vi "ToggleIndicator.vi"(11 "cClimbWeight":bool) -> (2 "True":bool, 3 "False":bool)   [LabVIEW 2013]
uses:
  ToggleStates.ctl
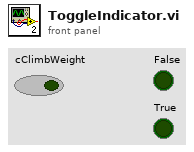
[diagram p1: front panel]
types:
  T1 = typedef "ToggleStates.ctl" = enum16{"Retract2", "Actuate1", "Actuate2", "Retract1"}
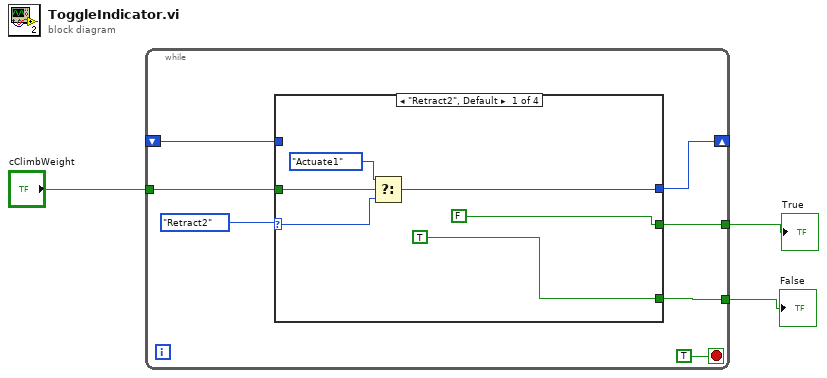
[diagram p0: block diagram]
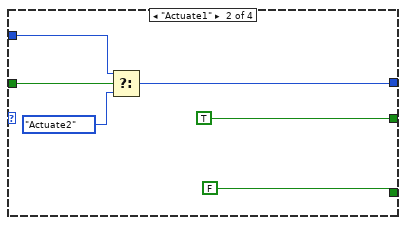
[diagram p2: hidden frame]
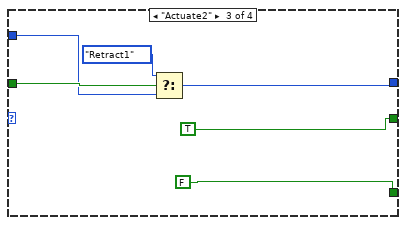
[diagram p3: hidden frame]
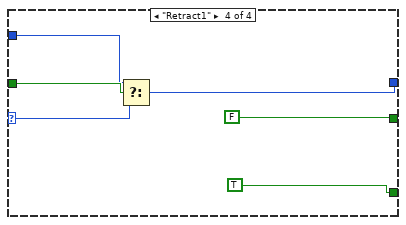
[diagram p4: hidden frame]
diagram:
  n1 = while {
    tunnel: "cClimbWeight" -> [w8]
    shift-right: [w7] -> _
    shift-left: _ -> [w6]
    tunnel: [w5] -> w2
    tunnel: [w4] -> w1
    stop <- TRUE stop-if-true
    n2 = case shown="\"Retract2\", Default" ToggleStates."Retract2" ("Enum") {
      selector: ToggleStates."Retract2" ("Enum") -> [w15 _ _ w29]
      tunnel: w8 -> [w16 w22 w28 w32]
      tunnel: [w13 w20 w23 w30] -> w7
      tunnel: w6 -> [_ w19 w25 w31]
      tunnel: [FALSE TRUE TRUE FALSE] -> w5
      tunnel: [TRUE FALSE FALSE TRUE] -> w4
      frame "Retract2", Default {
        n3 = Select(t=ToggleStates."Actuate1" ("Enum"), s=w16, f=w15) -> (s? t:f=w13:T1)
      }
      frame "Actuate1" {
        n4 = Select(t=w19, s=w22, f=ToggleStates."Actuate2" ("Enum")) -> (s? t:f=w20:T1)
      }
      frame "Actuate2" {
        n5 = Select(t=ToggleStates."Retract1" ("Enum"), s=w28, f=w25) -> (s? t:f=w23:T1)
      }
      frame "Retract1" {
        n6 = Select(t=w31, s=w32, f=w29) -> (s? t:f=w30:T1)
      }
    }
  }
  "True" <- w2
  "False" <- w1
